vi "6713_Blue_MOT_write_waveform_2015.10.19.vi"(8 "Error In":errorcluster, 9 "Control Reference \nCluster Input":T1, 11 "6713 Blue MOT":T2={"Active Device"="6229_Green_Lattice", "Active Channels"=[TRUE, TRUE, TRUE, TRUE, FALSE, FALSE, FALSE, FALSE], "Waveform Parameters"=[[{"Constant"=0.0, "Nickname"="", "Conversion"=enum."B Field Grad (G/cm)"}, {"Constant"=0.0, "Nickname"="", "Conversion"=enum."B Field Grad (G/cm)"}, {"Constant"=0.0, "Nickname"="", "Conversion"=enum."B Field Grad (G/cm)"}, {"Constant"=0.0, "Nickname"="", "Conversion"=enum."B Field Grad (G/cm)"}, {"Constant"=0.0, "Nickname"="", "Conversion"=enum."B Field Grad (G/cm)"}, {"Constant"=0.0, "Nickname"="", "Conversion"=enum."B Field Grad (G/cm)"}], [{"Constant"=0.0, "Nickname"="", "Conversion"=enum."B Field Grad (G/cm)"}, {"Constant"=0.0, "Nickname"="", "Conversion"=enum."B Field Grad (G/cm)"}, {"Constant"=0.0, "Nickname"="", "Conversion"=enum."B Field Grad (G/cm)"}, {"Constant"=0.0, "Nickname"="", "Conversion"=enum."B Field Grad (G/cm)"}, {"Constant"=0.0, "Nickname"="", "Conversion"=enum."B Field Grad (G/cm)"}, {"Constant"=0.0, "Nickname"="", "Conversion"=enum."B Field Grad (G/cm)"}], [{"Constant"=0.0, "Nickname"="", "Conversion"=enum."B Field Grad (G/cm)"}, {"Constant"=0.0, "Nickname"="", "Conversion"=enum."B Field Grad (G/cm)"}, {"Constant"=0.0, "Nickname"="", "Conversion"=enum."B Field Grad (G/cm)"}, {"Constant"=0.0, "Nickname"="", "Conversion"=enum."B Field Grad (G/cm)"}, {"Constant"=0.0, "Nickname"="", "Conversion"=enum."B Field Grad (G/cm)"}, {"Constant"=0.0, "Nickname"="", "Conversion"=enum."B Field Grad (G/cm)"}], [{"Constant"=0.0, "Nickname"="", "Conversion"=enum."B Field Grad (G/cm)"}, {"Constant"=0.0, "Nickname"="", "Conversion"=enum."B Field Grad (G/cm)"}, {"Constant"=0.0, "Nickname"="", "Conversion"=enum."B Field Grad (G/cm)"}, {"Constant"=0.0, "Nickname"="", "Conversion"=enum."B Field Grad (G/cm)"}, {"Constant"=0.0, "Nickname"="", "Conversion"=enum."B Field Grad (G/cm)"}, {"Constant"=0.0, "Nickname"="", "Conversion"=enum."B Field Grad (G/cm)"}], [{"Constant"=0.0, "Nickname"="", "Conversion"=enum."B Field Grad (G/cm)"}, {"Constant"=0.0, "Nickname"="", "Conversion"=enum."B Field Grad (G/cm)"}, {"Constant"=0.0, "Nickname"="", "Conversion"=enum."B Field Grad (G/cm)"}, {"Constant"=0.0, "Nickname"="", "Conversion"=enum."B Field Grad (G/cm)"}, {"Constant"=0.0, "Nickname"="", "Conversion"=enum."B Field Grad (G/cm)"}, {"Constant"=0.0, "Nickname"="", "Conversion"=enum."B Field Grad (G/cm)"}], [{"Constant"=0.0, "Nickname"="", "Conversion"=enum."B Field Grad (G/cm)"}, {"Constant"=0.0, "Nickname"="", "Conversion"=enum."B Field Grad (G/cm)"}, {"Constant"=0.0, "Nickname"="", "Conversion"=enum."B Field Grad (G/cm)"}, {"Constant"=0.0, "Nickname"="", "Conversion"=enum."B Field Grad (G/cm)"}, {"Constant"=0.0, "Nickname"="", "Conversion"=enum."B Field Grad (G/cm)"}, {"Constant"=0.0, "Nickname"="", "Conversion"=enum."B Field Grad (G/cm)"}], [{"Constant"=0.0, "Nickname"="", "Conversion"=enum."B Field Grad (G/cm)"}, {"Constant"=0.0, "Nickname"="", "Conversion"=enum."B Field Grad (G/cm)"}, {"Constant"=0.0, "Nickname"="", "Conversion"=enum."B Field Grad (G/cm)"}, {"Constant"=0.0, "Nickname"="", "Conversion"=enum."B Field Grad (G/cm)"}, {"Constant"=0.0, "Nickname"="", "Conversion"=enum."B Field Grad (G/cm)"}, {"Constant"=0.0, "Nickname"="", "Conversion"=enum."B Field Grad (G/cm)"}], [{"Constant"=0.0, "Nickname"="", "Conversion"=enum."B Field Grad (G/cm)"}, {"Constant"=0.0, "Nickname"="", "Conversion"=enum."B Field Grad (G/cm)"}, {"Constant"=0.0, "Nickname"="", "Conversion"=enum."B Field Grad (G/cm)"}, {"Constant"=0.0, "Nickname"="", "Conversion"=enum."B Field Grad (G/cm)"}, {"Constant"=0.0, "Nickname"="", "Conversion"=enum."B Field Grad (G/cm)"}, {"Constant"=0.0, "Nickname"="", "Conversion"=enum."B Field Grad (G/cm)"}]], "Active Phases"=[TRUE, FALSE, FALSE, FALSE, FALSE, FALSE], "Phase Times"=[1.0, 0.1, 0.1], "Trigger Channel"="/6229_Green_Lattice/PFI0", "FIFO Buffer Size"=8191.0, "6713_ch_labels"={"Array"=["", "", "", "", "", "", "", "", "", "", "", "", "", "", "", "", "", "", "", "", " ", "", "", ""], "PB_0_Ch_Labels\n"=["0", "1", "2", "3", "4", "5", "6", "7", "8", "9", "10", "11", "12", "13", "14", "15", "16", "17", "18", "19", "20", "21", "22", "23"]}} {"Phase Times" format="%.3f"}) -> (0 "error out":errorcluster, 2 "counter task out":refnum<k21>, 3 "waveform task out":refnum<k21>)   [LabVIEW 2016]
uses:
  Controls/6713/6713_waveform_generation.ctl
  Controls/6713/6713_waveform_parameter_array.ctl
  Controls/6713/6713_static_waveform_item.ctl
  6733_Red_MOT/Neutral_voltage_conversion_control.ctl
  Controls/6713/6713_ch_labels.ctl
  6733 arb waveforms/Control 1.ctl
  <vilib>/DAQmx/write.llb/DAQmx Write (Analog 1D DBL NChan 1Samp).vi
  <vilib>/DAQmx/write.llb/DAQmx Write (Analog 1D Wfm NChan NSamp).vi
  <vilib>/DAQmx/create/channels.llb/DAQmx Create Channel (AO-Voltage-Basic).vi
  <vilib>/DAQmx/miscellaneous.llb/DAQmx Fill In Error Info.vi
  <vilib>/Waveform/WDTOps.llb/WDT Append Waveforms DBL.vi
  <vilib>/Waveform/WDTOps.llb/WDT Scale Delta t DBL.vi
  <vilib>/DAQmx/configure/timing.llb/DAQmx Timing (Sample Clock).vi
  <vilib>/DAQmx/create/channels.llb/DAQmx Create Channel (CO-Pulse Generation-Frequency).vi
  <vilib>/DAQmx/configure/timing.llb/DAQmx Timing (Implicit).vi
  <vilib>/DAQmx/configure/trigger.llb/DAQmx Start Trigger (Digital Edge).vi
  <resource>/objmgr/daqmx.rc
panel:
  out "Total Time":dbl
  out "Sample Rate":dbl
  out "Waveforms":waveform(dbl)[](array[waveform])
  out "Max Sample Rate":dbl=1000000.0
  out "# Inactive Channels":i32
  out "# Active Channels":i16
  out "Inactive Channels":tag[](array[tag])
  out "Active Channels":tag[](array[tag])
  out "Samples Written":dbl
  out "Voltage Maximum":dbl
  out "Voltage Minimum":dbl
  out "AO.PhysicalChans":tag[](array[tag])
  out "Active Device":tag
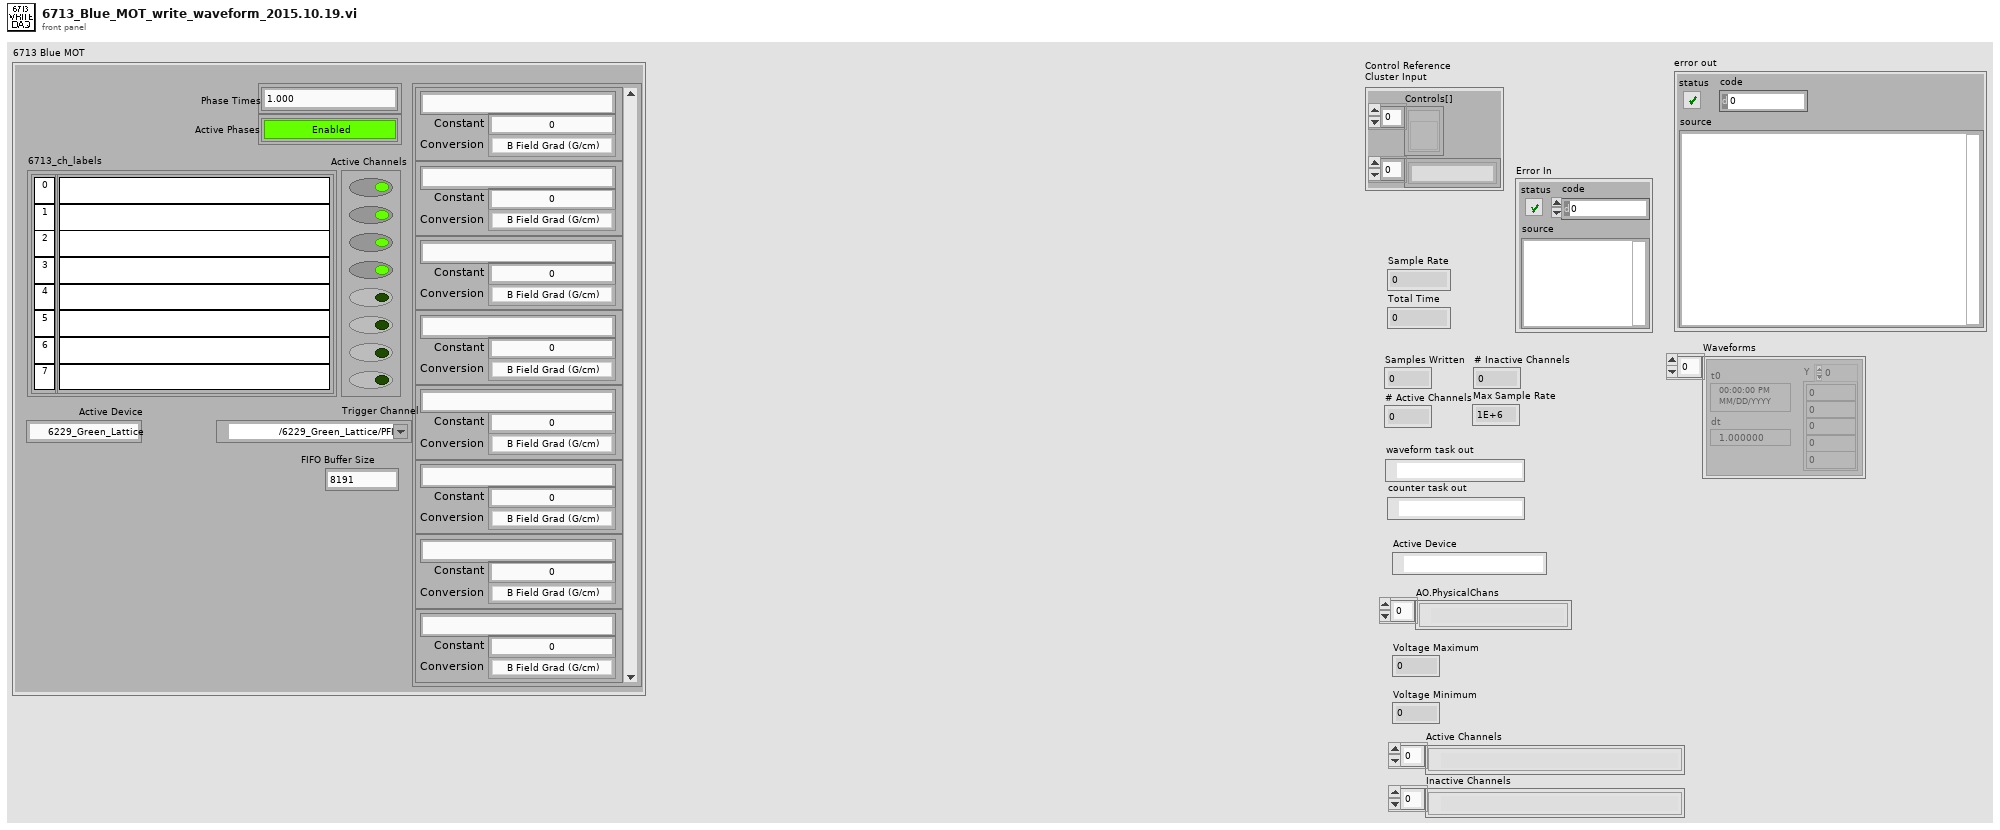
[diagram p1: front panel]
types:
  T1 = cluster{"Controls[]":refnum<vi>[], "Control Names":string[]}
  T2 = typedef "6713_waveform_generation.ctl" = cluster{"Active Device":string, "Active Channels":bool[], "Waveform Parameters":T3, "Active Phases":bool[], "Phase Times":dbl[], "Trigger Channel":tag, "FIFO Buffer Size":dbl, "6713_ch_labels":T6}
  T3 = typedef "6713_waveform_parameter_array.ctl" = T4[][]
  T4 = typedef "6713_static_waveform_item.ctl" = cluster{"Constant":dbl, "Nickname":string, "Conversion":T5}
  T5 = typedef "Neutral_voltage_conversion_control.ctl" = enum16{"Volts", "B Field Grad (G/cm)", "Red Boson Cntr Freq (MHz)", "Red Boson Dither Amp (kHz)", "Red Boson Power (mW)", "Red 87 Trap Cntr Freq (MHz)", "Red 87 Trap Dither Amp (kHz)", "Red 87 Trap Power (mW)", "Red 87 Stir Cntr Freq (MHz)", "Red 87 Stir Dither Amp (kHz)", "Red 87 Stir Power (mW)", "ODT Sheet Trap Power (W)", "ODT Loading Trap Power (W)"}
  T6 = typedef "6713_ch_labels.ctl" = cluster{"Array":string[], "PB_0_Ch_Labels\n":string[]}
  T7 = typedef "Control 1.ctl" = enum16{"Initialize", "Get Device Information", "Get Active/Inactive Channels", "Maximize Samples / Channel", "Calculate Waveforms", "Check for Problems", "Update Front Panel", "Clear Old Tasks", "Write Initialization to Cards", "Write Waveform to Cards"}
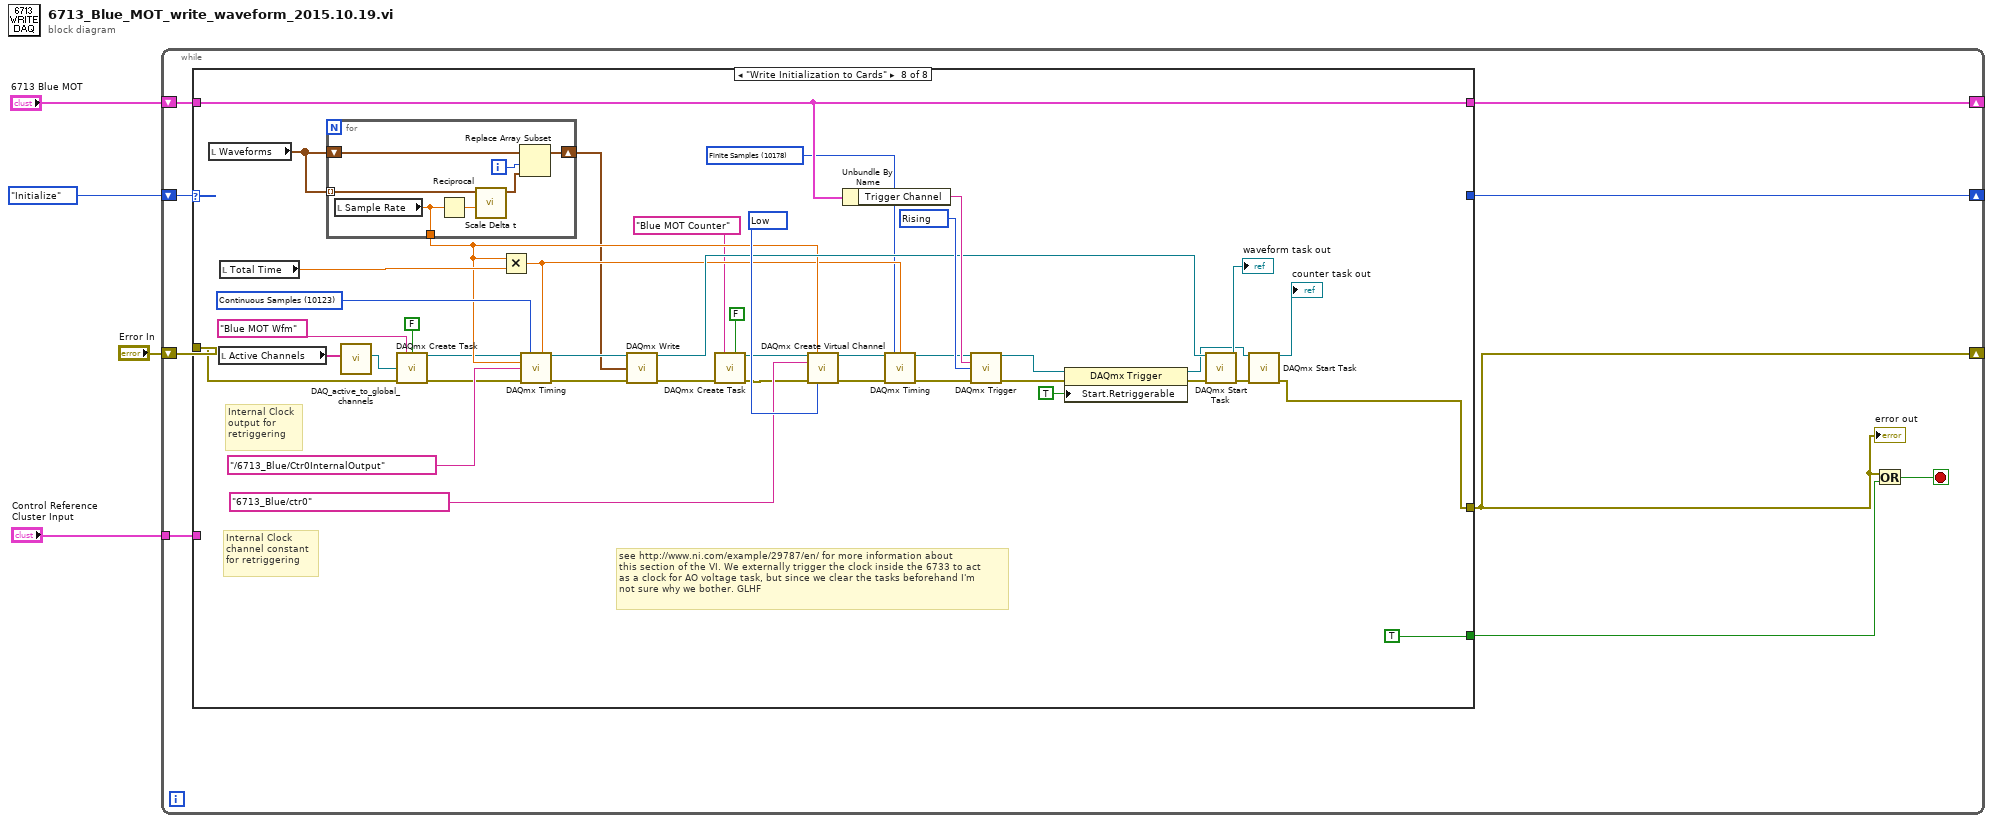
[diagram p0: block diagram]
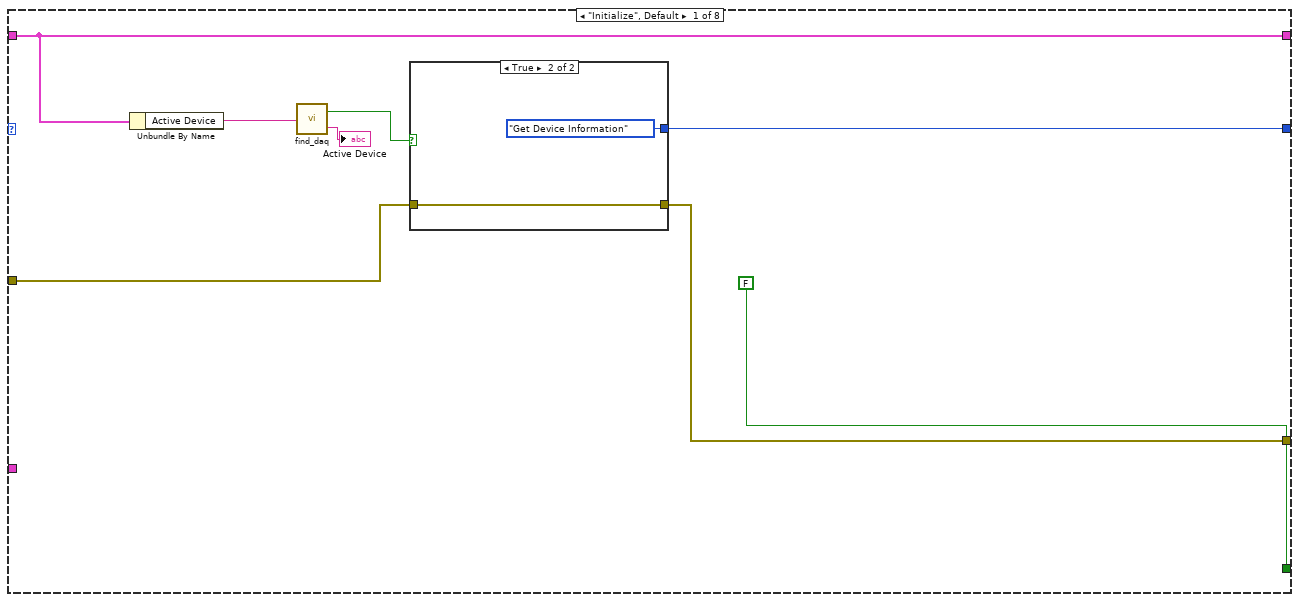
[diagram p2: hidden frame]
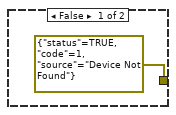
[diagram p3: hidden frame]
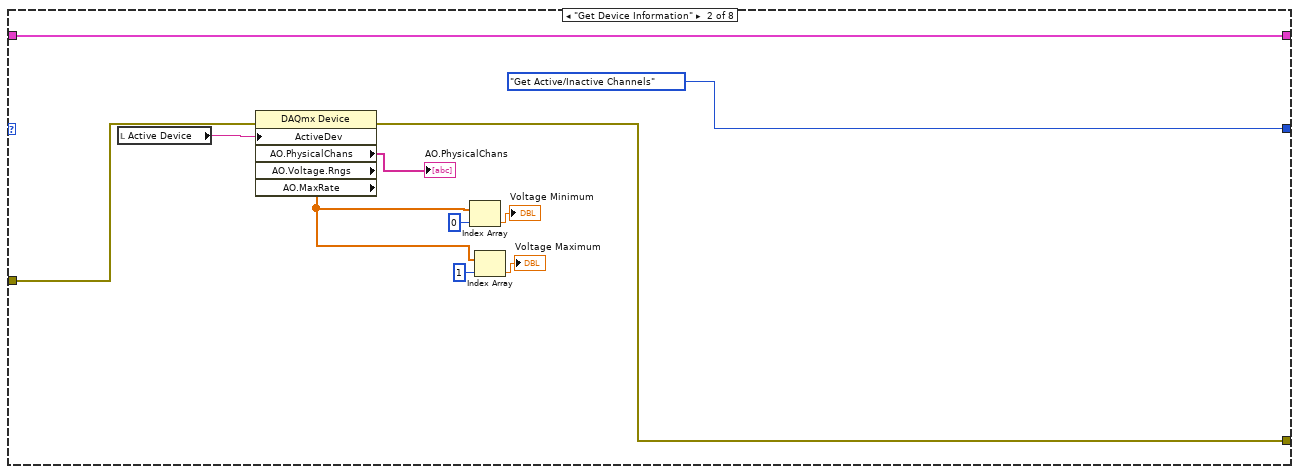
[diagram p4: hidden frame]
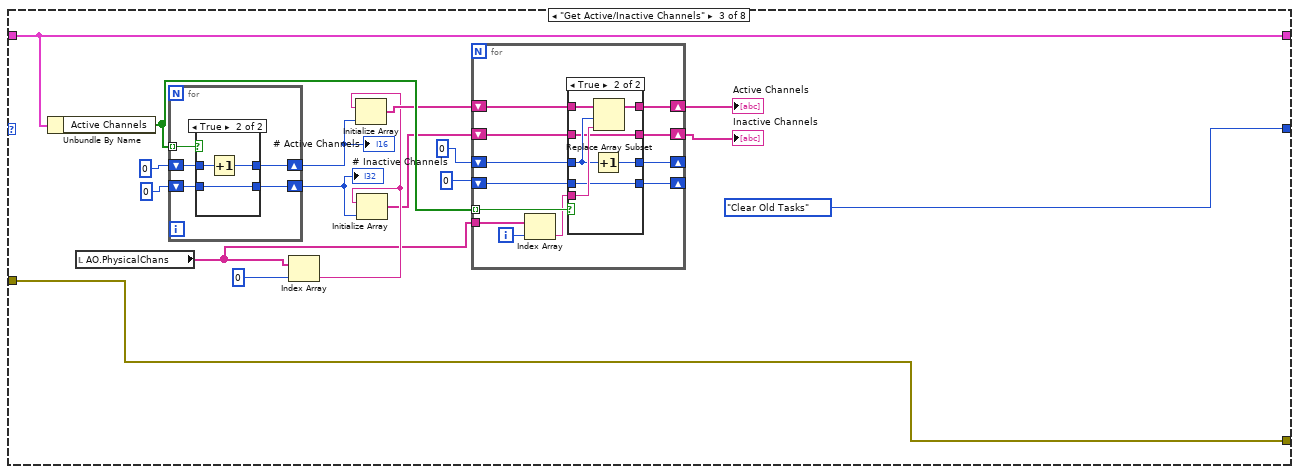
[diagram p5: hidden frame]
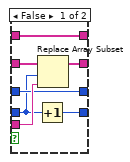
[diagram p6: hidden frame]
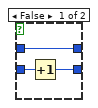
[diagram p7: hidden frame]
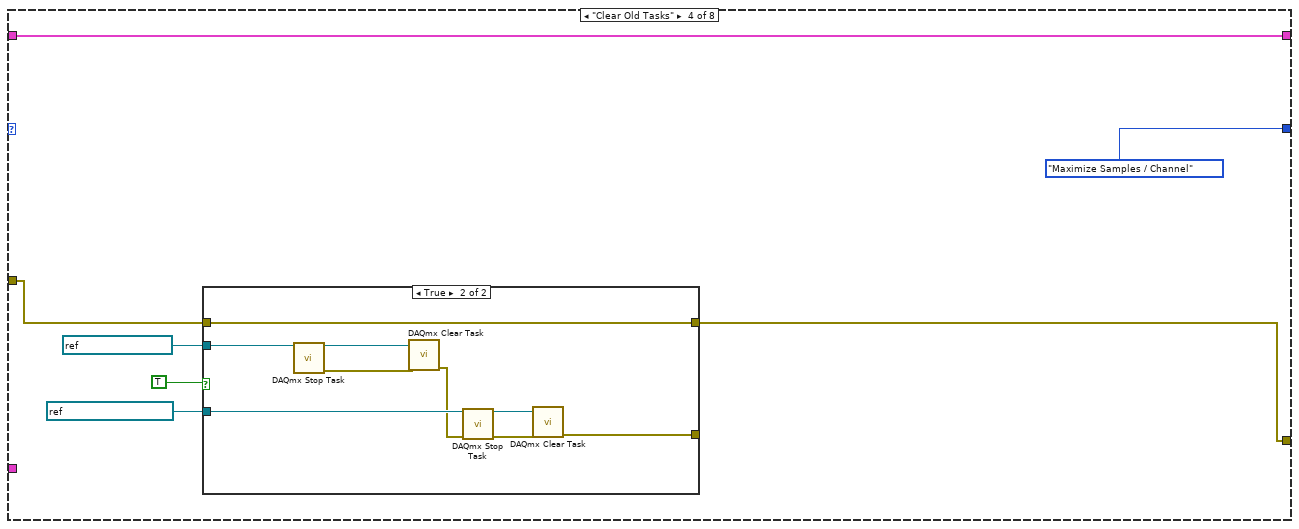
[diagram p8: hidden frame]
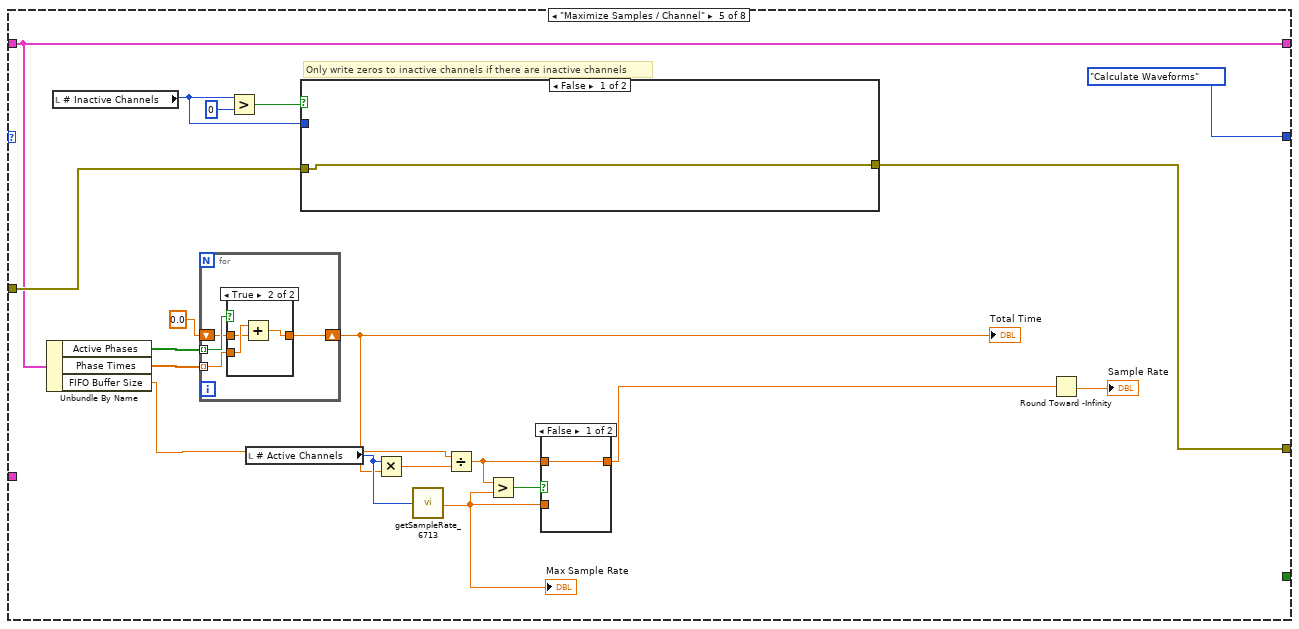
[diagram p10: hidden frame]
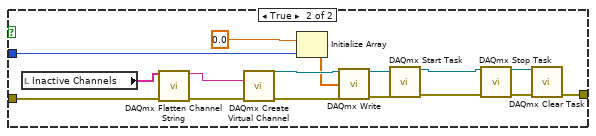
[diagram p11: hidden frame]
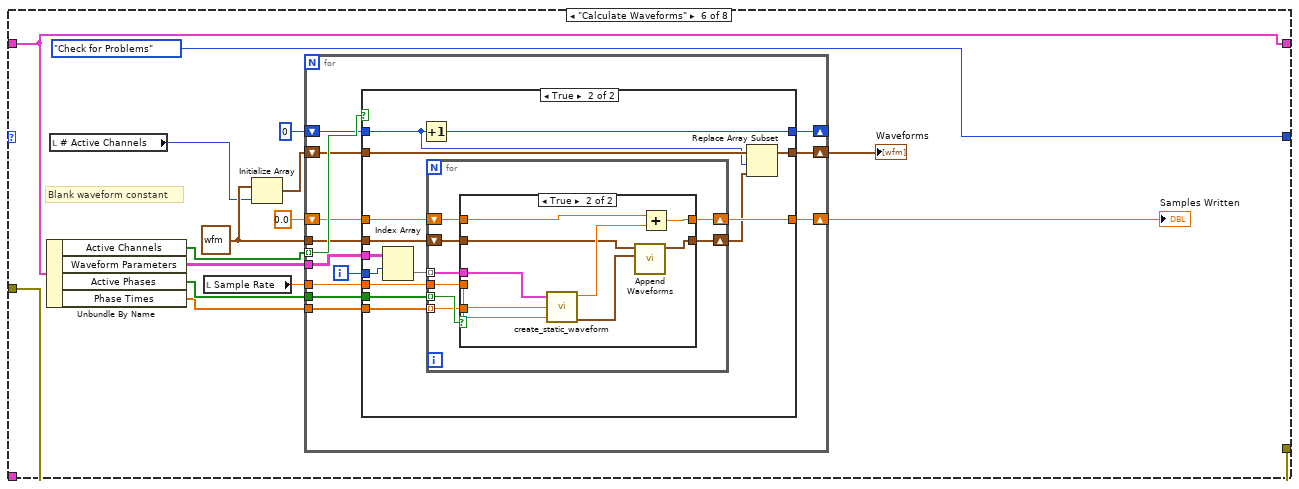
[diagram p14: hidden frame]
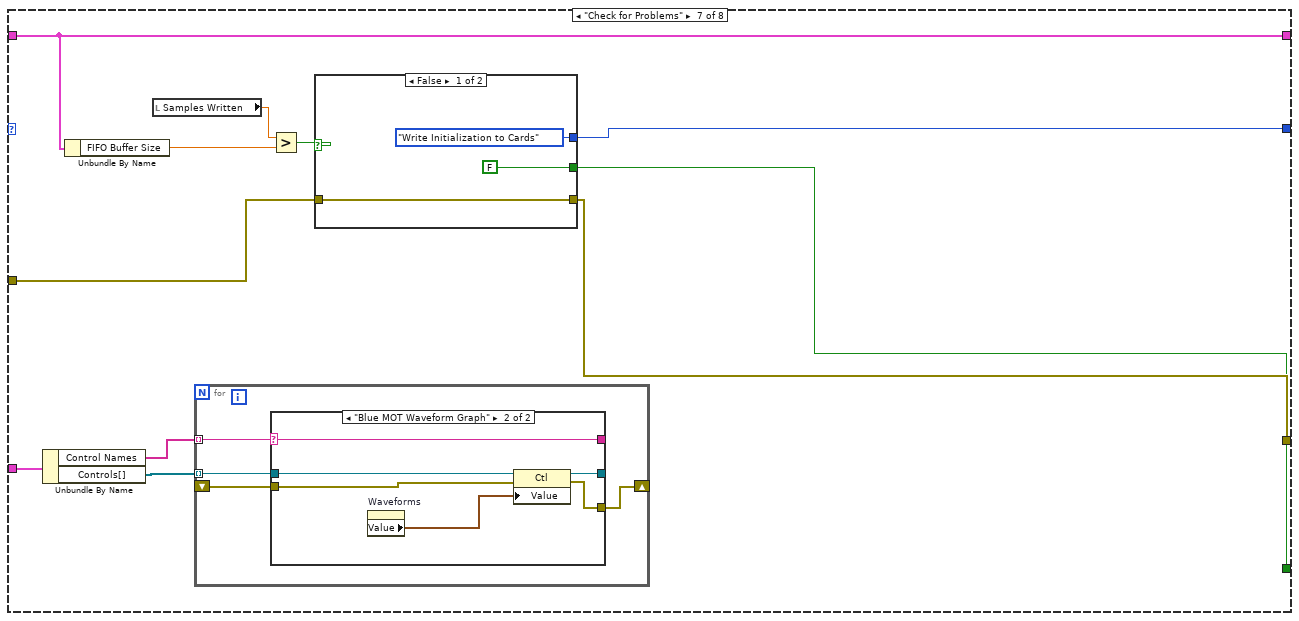
[diagram p17: hidden frame]
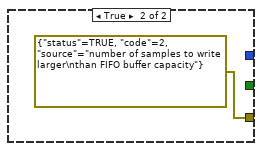
[diagram p19: hidden frame]
diagram:
  n1 = while {
    shift-right: [w9] -> _
    shift-left: "Error In" -> [w11]
    shift-right: [w10] -> _
    shift-left: Control_1."Initialize" -> [w13]
    shift-right: [w7] -> _
    shift-left: "6713 Blue MOT" -> [w12]
    tunnel: "Control Reference \nCluster Input" -> [w5]
    stop <- w8 stop-if-true
    n2 = case shown="\"Write Initialization to Cards\"" w13 {
      tunnel: w12 -> [w15 w35 w39 w92 w111 w163 w220 w284]
      tunnel: [w18 w27 w50 w95 w124 w166 w225 w263] -> w9
      tunnel: w11 -> [w17 w34 w50 w94 w125 w166 w226 w258]
      tunnel: [w16 Control_1."Get Active/Inactive Channels" Control_1."Clear Old Tasks" Control_1."Maximize Samples / Channel" Control_1."Calculate Waveforms" Control_1."Check for Problems" w224 _] -> w10
      tunnel: [w15 w35 w39 w92 w111 w163 w220 w284] -> w7
      tunnel: [FALSE ("y") _ _ _ _ _ w223 TRUE ("y")] -> w6
      tunnel: w5 -> [_ _ _ _ _ _ w217 _]
      frame "Initialize", Default {
        n3 = Unbundle By Name(w15) -> ("Active Device"=w21:string)
        n4 = call "find_daq.vi"("Device Name"=w21) -> ("Device Present"=w19:bool, "DAQmx Device Name"=→"Active Device":tag)
        n5 = case shown="True" w19 {
          tunnel: [errorcluster {"status"=TRUE, "code"=1, "source"="Device Not Found"} ("error in (no error)") w24] -> w18
          tunnel: w17 -> [_ w24]
          tunnel: [_ Control_1."Get Device Information"] -> w16
          frame False {
          }
          frame True {
          }
        }
      }
      frame "Get Device Information" {
        n6 = local read "Active Device"() -> (w25:tag)
        n7 = property class="DAQmx Device" props=["ActiveDev", "AO.PhysicalChans", "AO.Voltage.Rngs", "AO.MaxRate"](error in=w34, "ActiveDev"=w25) -> (error out=w27:errorcluster, "AO.PhysicalChans"=→"AO.PhysicalChans":tag[], "AO.Voltage.Rngs"=w29:dbl[])  [unwired: 1 in, 2 out]
        n8 = Index Array(array=w29, index=0) -> (element=→"Voltage Minimum":dbl)
        n9 = Index Array(array=w29, index=1) -> (element=→"Voltage Maximum":dbl)
      }
      frame "Get Active/Inactive Channels" {
        n10 = Unbundle By Name(w39) -> ("Active Channels"=w49:bool[])
        n11 = local read "AO.PhysicalChans"() -> (w43:tag[])
        n12 = for {
          shift-right: [w83] -> w48
          shift-left: i16 0 -> [w82]
          shift-right: [w81] -> w47
          shift-left: 0 -> [w80]
          tunnel: w49 -> [w79] mode=indexing
          n13 = case shown="True" w79 {
            tunnel: [w84 w89] -> w83
            tunnel: w82 -> [w84 w88]
            tunnel: [w86 w87] -> w81
            tunnel: w80 -> [w85 w87]
            frame False {
              n14 = Increment(x=w85) -> (x+1=w86:i32)
            }
            frame True {
              n15 = Increment(x=w88) -> (x+1=w89:i16)
            }
          }
        }
        "# Active Channels" <- w48
        "# Inactive Channels" <- w47
        n16 = Index Array(array=w43, index=0) -> (element=w44:tag)
        n17 = Initialize Array(w44, w48) -> (w46:tag[])
        n18 = Initialize Array(w44, w47) -> (w42:tag[])
        n19 = for {
          tunnel: w49 -> [w64] mode=indexing
          shift-right: [w61] -> w38
          shift-left: w46 -> [w62]
          tunnel: w43 -> [w59]
          shift-right: [w57] -> w37
          shift-left: w42 -> [w58]
          shift-right: [w55] -> _
          shift-left: 0 ("index") -> [w56]
          shift-right: [w53] -> _
          shift-left: 0 ("index") -> [w54]
          i -> [w63]
          n20 = Index Array(array=w59, index=w63) -> (element=w60:tag)
          n21 = case shown="True" w64 {
            tunnel: w62 -> [w65 w78]
            tunnel: [w65 w77] -> w61
            tunnel: w60 -> [w71 w76]
            tunnel: w58 -> [w70 w72]
            tunnel: [w69 w72] -> w57
            tunnel: w56 -> [w68 w75]
            tunnel: [w68 w74] -> w55
            tunnel: w54 -> [w67 w73]
            tunnel: [w66 w73] -> w53
            frame False {
              n22 = Increment(x=w67) -> (x+1=w66:i32)
              n23 = Replace Array Subset(array=w70, new element=w71, index=w67) -> (w69:tag[])
            }
            frame True {
              n24 = Increment(x=w75) -> (x+1=w74:i32)
              n25 = Replace Array Subset(array=w78, new element=w76, index=w75) -> (w77:tag[])
            }
          }
        }
        "Active Channels" <- w38
        "Inactive Channels" <- w37
      }
      frame "Clear Old Tasks" {
        n26 = case shown="True" TRUE {
          tunnel: refnum<k21> "Blue MOT Wfm" ("Waveform Task In") -> [_ w106]
          tunnel: refnum<k21> "Blue MOT Counter" ("Control Task In") -> [_ w104]
          tunnel: [w97 w102] -> w95
          tunnel: w94 -> [w97 w102]
          tunnel: [_ w98] -> _
          frame False {
          }
          frame True {
            n27 = call <vilib>:"DAQmx Stop Task.vi"("task/channels in"=w106) -> ("task out"=w105:refnum<k21>, "error out"=w101:errorcluster)  [unwired: 13 in]
            n28 = call <vilib>:"DAQmx Clear Task.vi"("task in"=w105, "error in"=w101) -> ("error out"=w100:errorcluster)  [unwired: 13 in]
            n29 = call <vilib>:"DAQmx Stop Task.vi"("task/channels in"=w104, "error in"=w100) -> ("task out"=w103:refnum<k21>, "error out"=w99:errorcluster)  [unwired: 12 in]
            n30 = call <vilib>:"DAQmx Clear Task.vi"("task in"=w103, "error in"=w99) -> ("error out"=w98:errorcluster)  [unwired: 13 in]
          }
        }
      }
      frame "Maximize Samples / Channel" {
        # "Only write zeros to inactive channels if there are inactive channels"
        n31 = Unbundle By Name(w111) -> ("Active Phases"=w122:bool[], "Phase Times"=w121:dbl[], "FIFO Buffer Size"=w110:dbl)
        n32 = local read "# Inactive Channels"() -> (w109:i32)
        n33 = for {
          tunnel: w122 -> [w148] mode=indexing
          tunnel: w121 -> [w147] mode=indexing
          shift-right: [w145] -> w116
          shift-left: 0.0 -> [w146]
          n34 = case shown="True" w148 {
            tunnel: w147 -> [_ w152]
            tunnel: w146 -> [w149 w151]
            tunnel: [w149 w150] -> w145
            frame False {
            }
            frame True {
              n35 = Add(x=w152, y=w151) -> (x+y=w150:dbl)
            }
          }
        }
        "Total Time" <- w116
        n36 = Greater?(x=w109, y=0) -> (0:w108:bool)
        n37 = local read "# Active Channels"() -> (w117:i16)
        n38 = case shown="False" w108 {
          tunnel: w125 -> [w126 w140]
          tunnel: [w126 w130] -> w124
          tunnel: w109 -> [_ w127]
          frame False {
          }
          frame True {
            n39 = local read "Inactive Channels"() -> (w141:tag[])
            n40 = call <vilib>:"DAQmx Flatten Channel String.vi"("names in"=w141, "error in"=w140) -> ("names out"=w139:string, "error out"=w142:errorcluster)  [unwired: 12 in]
            n41 = call-poly <vilib>:"DAQmx Create Virtual Channel.vi"("physical channels"=w139, "error in"=w142) -> ("task out"=w138:refnum<k21>, "error out"=w137:errorcluster)  [unwired: 12 in]
            n42 = Initialize Array(0.0 ("element"), w127) -> (w133:dbl[])
            n43 = call-poly <vilib>:"DAQmx Write.vi"("task/channels in"=w138, "data"=w133, "error in"=w137) -> ("task out"=w135:refnum<k21>, "error out"=w136:errorcluster)  [unwired: 10 in, 1 out]
            n44 = call <vilib>:"DAQmx Start Task.vi"("task/channels in"=w135, "error in"=w136) -> ("task out"=w128:refnum<k21>, "error out"=w129:errorcluster)  [unwired: 12 in]
            n45 = call <vilib>:"DAQmx Stop Task.vi"("task/channels in"=w128, "error in"=w129) -> ("task out"=w132:refnum<k21>, "error out"=w131:errorcluster)  [unwired: 12 in]
            n46 = call <vilib>:"DAQmx Clear Task.vi"("task in"=w132, "error in"=w131) -> ("error out"=w130:errorcluster)  [unwired: 13 in]
          }
        }
        n47 = Multiply(x=w117, y=w116) -> (x*y=w118:dbl)
        n48 = call "getSampleRate_6713.vi"("Number of active channels"=w117) -> ("Sample Rate"=w115:dbl)
        "Max Sample Rate" <- w115
        n49 = Divide(x=w110, y=w118) -> (x/y=w114:dbl)
        n50 = Greater?(x=w114, y=w115) -> (0:w119:bool)
        n51 = case shown="False" w119 {
          tunnel: [w143 w144] -> w112
          tunnel: w115 -> [_ w144]
          tunnel: w114 -> [w143 _]
          frame False {
          }
          frame True {
          }
        }
        n52 = Round Toward -Infinity(1:w112) -> (0:→"Sample Rate":dbl)
      }
      frame "Calculate Waveforms" {
        w160 = waveform(dbl) {"t0"=timestamp(0 s since 1904-01-01), "dt"=1.0, "Y"=[]}
        # "Blank waveform constant"
        n53 = Unbundle By Name(w163) -> ("Active Channels"=w155:bool[], "Waveform Parameters"=w167:T3, "Active Phases"=w161:bool[], "Phase Times"=w156:dbl[])
        n54 = local read "# Active Channels"() -> (w153:i16)
        n55 = local read "Sample Rate"() -> (w154:dbl)
        n56 = Initialize Array(w160, w153) -> (w158:waveform(dbl)[])
        n57 = for {
          tunnel: w155 -> [w180] mode=indexing
          tunnel: w167 -> [w178]
          shift-right: [w177] -> w165
          shift-left: 0.0 -> [w176]
          tunnel: w161 -> [w175]
          tunnel: w160 -> [w174]
          shift-right: [w172] -> _
          shift-left: 0 -> [w173]
          shift-right: [w170] -> w157
          shift-left: w158 -> [w171]
          tunnel: w156 -> [w169]
          tunnel: w154 -> [w168]
          i -> [w179]
          n58 = case shown="True" w180 {
            tunnel: w179 -> [_ w197]
            tunnel: w178 -> [_ w196]
            tunnel: [w183 w195] -> w177
            tunnel: w176 -> [w183 w194]
            tunnel: w175 -> [_ w192]
            tunnel: w174 -> [_ w191]
            tunnel: w173 -> [w182 w188]
            tunnel: [w182 w190] -> w172
            tunnel: w171 -> [w181 w189]
            tunnel: [w181 w186] -> w170
            tunnel: w169 -> [_ w185]
            tunnel: w168 -> [_ w184]
            frame False {
            }
            frame True {
              n59 = Index Array(array=w196, index (row)=w197) -> (element=w193:T4[])  [unwired: 1 in]
              n60 = Increment(x=w188) -> (x+1=w190:i32)
              n61 = for {
                shift-right: [w205] -> w195
                shift-left: w194 -> [w204]
                tunnel: w193 -> [w203] mode=indexing
                shift-right: [w201] -> w187
                shift-left: w191 -> [w202]
                tunnel: w192 -> [w200] mode=indexing
                tunnel: w185 -> [w199] mode=indexing
                tunnel: w184 -> [w198]
                n62 = case shown="True" w200 {
                  tunnel: [w207 w215] -> w205
                  tunnel: w204 -> [w207 w214]
                  tunnel: w203 -> [_ w210]
                  tunnel: w202 -> [w206 w212]
                  tunnel: [w206 w211] -> w201
                  tunnel: w199 -> [_ w209]
                  tunnel: w198 -> [_ w208]
                  frame False {
                  }
                  frame True {
                    n63 = call "create_static_waveform.vi"("Waveform Parameters"=w210, "Sample rate"=w208, "Time"=w209) -> ("Samples to Write"=w216:dbl, "output waveform"=w213:waveform(dbl))  [unwired: 1 in, 1 out]
                    n64 = call-poly <vilib>:"Append Waveforms.vi"("waveform B"=w213, "waveform A"=w212) -> ("waveform out"=w211:waveform(dbl))  [unwired: 8 in, 1 out]
                    n65 = Add(x=w214, y=w216) -> (x+y=w215:dbl)
                  }
                }
              }
              n66 = Replace Array Subset(array=w189, new element=w187, index=w188) -> (w186:waveform(dbl)[])
            }
          }
        }
        "Samples Written" <- w165
        "Waveforms" <- w157
      }
      frame "Check for Problems" {
        n67 = Unbundle By Name(w217) -> ("Control Names"=w219:string[], "Controls[]"=w218:refnum<vi>[])
        n68 = Unbundle By Name(w220) -> ("FIFO Buffer Size"=w221:dbl)
        n69 = local read "Samples Written"() -> (w222:dbl)
        n70 = for {
          tunnel: w219 -> [w231] mode=indexing
          shift-right: [w228] -> _
          shift-left: _ -> [w229]
          tunnel: w218 -> [w230] mode=indexing
          n71 = case shown="\"Blue MOT Waveform Graph\"" w231 {
            selector: w231 -> [w234 w240]
            tunnel: w230 -> [w233 w237]
            tunnel: [w234 w240] -> _
            tunnel: [w233 w236] -> _
            tunnel: w229 -> [w232 w239]
            tunnel: [w232 w238] -> w228
            frame "False", Default {
            }
            frame "Blue MOT Waveform Graph" {
              n72 = property on="Waveforms" class="Arr (strict)"() -> ("Value"=w235:waveform(dbl)[])  [unwired: 2 in, 2 out]
              n73 = property class="Ctl"(reference=w237, error in=w239, "Value"=w235) -> (reference out=w236:refnum<vi>, error out=w238:errorcluster)
            }
          }
        }
        n74 = Greater?(x=w222, y=w221) -> (0:w227:bool)
        n75 = case shown="False" w227 {
          tunnel: w226 -> [w243 _]
          tunnel: [w243 errorcluster {"status"=TRUE, "code"=2, "source"="number of samples to write larger\nthan FIFO buffer capacity"} ("error in (no error)")] -> w225
          tunnel: [Control_1."Write Initialization to Cards" _] -> w224
          tunnel: [FALSE ("y") _] -> w223
          frame False {
          }
          frame True {
          }
        }
      }
      frame "Write Initialization to Cards" {
        w246 = 10178 items=["Finite Samples"=10178, "Continuous Samples"=10123, "Hardware Timed Single Point"=12522] ("sample mode")
        w275 = 10280 items=["Rising"=10280, "Falling"=10171] ("edge")
        w279 = 10123 items=["Finite Samples"=10178, "Continuous Samples"=10123, "Hardware Timed Single Point"=12522] ("sample mode")
        w283 = 10214 items=["High"=10192, "Low"=10214] ("idle state")
        # "see http://www.ni.com/example/29787/en/ for more information about\nthis section of the VI. We externally trigger the clock inside the 6733 to act\nas a clock for AO voltage task, but since we clear the tasks beforehand I'm\nnot sure why we bother. GLHF"
        # "Internal Clock\noutput for\nretriggering"
        # "Internal Clock\nchannel constant\nfor retriggering"
        n76 = local read "Waveforms"() -> (w285:waveform(dbl)[])
        n77 = local read "Active Channels"() -> (w259:tag[])
        n78 = local read "Total Time"() -> (w280:dbl)
        n79 = for {
          tunnel: w285 -> [w293] mode=indexing
          shift-right: [w287] -> w245
          shift-left: w285 -> [w289]
          tunnel: [w288] -> w266
          i -> [w291]
          n80 = local read "Sample Rate"() -> (w288:dbl)
          n81 = Reciprocal(x=w288) -> (1/x=w292:dbl)
          n82 = call-poly <vilib>:"Scale Delta t.vi"("scale factor"=w292, "waveform in"=w293) -> ("waveform out"=w290:waveform(dbl))  [unwired: 8 in, 1 out]
          n83 = Replace Array Subset(array=w289, new element=w290, index=w291) -> (w287:waveform(dbl)[])
        }
        n84 = call "DAQ_active_to_global_channels.vi"("Active Channels"=w259) -> ("Global Channels"=w256:refnum<k21>)  [unwired: 10 in]
        n85 = call <vilib>:"DAQmx Create Task.vi"("new task name"="Blue MOT Wfm", "auto cleanup"=FALSE, "global virtual channels"=w256, "error in"=w258) -> ("task out"=w254:refnum<k21>, "error out"=w257:errorcluster)  [unwired: 10 in]
        n86 = Multiply(x=w266, y=w280) -> (x*y=w260:dbl)
        n87 = call-poly <vilib>:"DAQmx Timing.vi"("task/channels in"=w254, "sample mode"=w279, "samples per channel"=w260, "rate"=w266, "source"=tag "/6713_Blue/Ctr0InternalOutput", "error in"=w257) -> ("task out"=w277:refnum<k21>, "error out"=w278:errorcluster)  [unwired: 8 in]
        n88 = call-poly <vilib>:"DAQmx Write.vi"("task/channels in"=w277, "data"=w245, "error in"=w278) -> ("task out"=w269:refnum<k21>, "error out"=w253:errorcluster)  [unwired: 10 in, 1 out]
        n89 = call <vilib>:"DAQmx Create Task.vi"("new task name"="Blue MOT Counter", "auto cleanup"=FALSE, "error in"=w253) -> ("task out"=w248:refnum<k21>, "error out"=w252:errorcluster)  [unwired: 11 in]
        n90 = call-poly <vilib>:"DAQmx Create Virtual Channel.vi"("task in"=w248, "frequency"=w266, "counter"=tag "6713_Blue/ctr0", "error in"=w252, "idle state"=w283) -> ("task out"=w282:refnum<k21>, "error out"=w281:errorcluster)  [unwired: 9 in]
        n91 = Unbundle By Name(w284) -> ("Trigger Channel"=w274:tag)
        n92 = call-poly <vilib>:"DAQmx Timing.vi"("task/channels in"=w282, "sample mode"=w246, "samples per channel"=w260, "error in"=w281) -> ("task out"=w273:refnum<k21>, "error out"=w276:errorcluster)  [unwired: 10 in]
        n93 = call-poly <vilib>:"DAQmx Trigger.vi"("task/channels in"=w273, "source"=w274, "edge"=w275, "error in"=w276) -> ("task out"=w271:refnum<k21>, "error out"=w272:errorcluster)  [unwired: 10 in]
        n94 = property class="DAQmx Trigger"(reference=w271, error in=w272, "Start.Retriggerable"=TRUE) -> (reference out=w247:refnum<k21>, error out=w268:errorcluster)
        n95 = call <vilib>:"DAQmx Start Task.vi"("task/channels in"=w269, "error in"=w268) -> ("task out"=→"waveform task out":refnum<k21>, "error out"=w267:errorcluster)  [unwired: 12 in]
        n96 = call <vilib>:"DAQmx Start Task.vi"("task/channels in"=w247, "error in"=w267) -> ("task out"=→"counter task out":refnum<k21>, "error out"=w263:errorcluster)  [unwired: 12 in]
      }
    }
    "error out" <- w9
    n97 = Or(x=w9, y=w6) -> (x .or. y?=w8:bool)
  }
